vi "Retro Normalize Coordinates.vi"(9 "Camera Type":T1, 10 "Scores":T4(array[cluster]), 11 "Image in":T5) -> (2 "Found Totes":T2(array[cluster]) {"Normalized Rect"."Numeric 5" format="%#_2g"; "Normalized Rect"."Numeric 3" format="%#_2g"; "Normalized Rect"."Numeric 2" format="%#_2g"; "Normalized Rect"."Numeric" format="%#_2g"}, 3 "Sorted Scores":T3(array[cluster]) {"Aspect Ratio" format="%#_3g"; "Area Score" format="%#_3g"; "X" format="%#_3g"; "Y" format="%#_3g"})   [LabVIEW 2025]
doc: "Normalize the rectangle and center so that they range from -1 to 1, left to right and bottom to top. This helps with producing joystick coordinates for driving the robot."
uses:
  <vilib>/vision/Image Controls.llb/IMAQ Image.ctl
  Camera Types.ctl
panel:
  # "Density Profile"
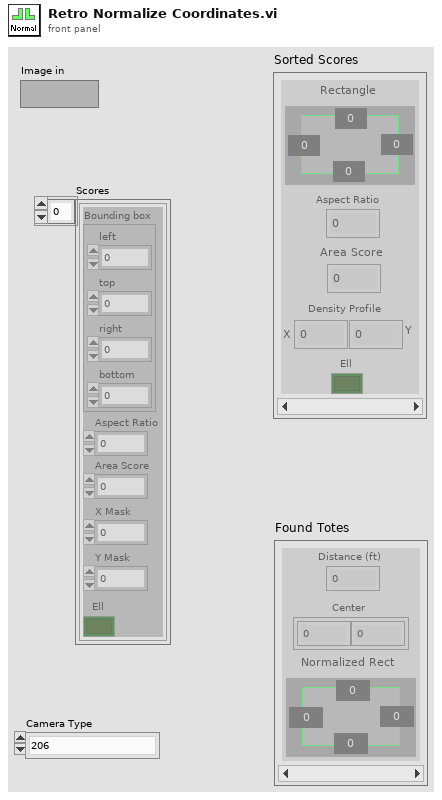
[diagram p1: front panel]
types:
  T1 = typedef "Camera Types.ctl" = enum16{"206", "1011", "1013", "MS HD3000 square", "MS HD3000 640x480"}
  T2 = cluster{"Distance (ft)":dbl, "Center":cluster{dbl, dbl}, "Normalized Rect":cluster{"Numeric":dbl, "Numeric 2":dbl, "Numeric 3":dbl, "Numeric 5":dbl}}[]
  T3 = cluster{"Rectangle":cluster{"Numeric":dbl, "Numeric 2":dbl, "Numeric 3":dbl, "Numeric 5":dbl}, "Aspect Ratio":dbl, "Area Score":dbl, "X":dbl, "Y":dbl, "Ell":bool}[]
  T4 = cluster{"Bounding box":cluster{"left":dbl, "top":dbl, "right":dbl, "bottom":dbl}, "Aspect Ratio":dbl, "Area Score":dbl, "X Mask":dbl, "Y Mask":dbl, "Ell":bool}[]
  T5 = typedef "IMAQ Image.ctl" = refnum<image>
  T6 = cluster{"left":dbl, "top":dbl, "right":dbl, "bottom":dbl}
  T7 = cluster{"X Resolution":i32, i32, "X Resolution":i32, i32}
  T8 = cluster{"Distance (ft)":dbl, cluster{dbl, dbl}, cluster{dbl, dbl, dbl, dbl}}
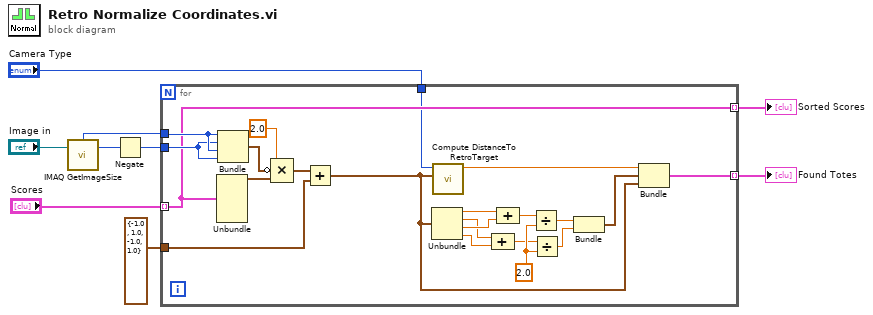
[diagram p0: block diagram]
diagram:
  n1 = call "IMAQ GetImageSize"("Image"="Image in") -> ("Y Resolution"=w7:i32, "X Resolution"=w8:i32)  [unwired: 3 in, 1 out]
  n2 = Negate(x=w7) -> (-x=w9:i32)
  n3 = for {
    tunnel: "Scores" -> [w14] mode=indexing
    tunnel: w9 -> [w30]
    tunnel: w8 -> [w31]
    tunnel: [w16] -> w4 mode=indexing
    tunnel: [w14] -> w1 mode=indexing
    tunnel: cluster{dbl, dbl, dbl, dbl} {-1.0, 1.0, -1.0, 1.0} ("y") -> [w13]
    tunnel: "Camera Type" -> [w11]
    w21 = 2.0
    n4 = Unbundle(w14) -> ("Bounding box"=w28:T6)  [unwired: 5 out]
    n5 = Bundle("X Resolution"=w31, w30, "X Resolution"=w31, w30) -> (w29:T7)  [unwired: 1 in]
    n6 = Compound Arithmetic op=MULTIPLY(2.0, invert w29, w28) -> (w27:cluster{dbl, dbl, dbl, dbl})
    n7 = Add(x=w27, y=w13) -> (x+y=w12:cluster{dbl, dbl, dbl, dbl})
    n8 = Unbundle(w12) -> (w25:dbl, w22:dbl, w24:dbl, w23:dbl)
    n9 = call "Compute DistanceTo RetroTarget.vi"("Norm Rect"=w12, "Camera Type"=w11) -> ("Distance (ft)"=w10:dbl)  [unwired: 9 in]
    n10 = Compound Arithmetic op=ADD(w22, w23) -> (w19:dbl)
    n11 = Compound Arithmetic op=ADD(w25, w24) -> (w20:dbl)
    n12 = Divide(x=w20, y=w21) -> (x/y=w18:dbl)
    n13 = Divide(x=w19, y=w21) -> (x/y=w17:dbl)
    n14 = Bundle(w18, w17) -> (w15:cluster{dbl, dbl})  [unwired: 1 in]
    n15 = Bundle("Distance (ft)"=w10, w15, w12) -> (w16:T8)  [unwired: 1 in]
  }
  "Sorted Scores" <- w1
  "Found Totes" <- w4
